vi "Get StartStop Status.vi"(8 "error in":errorcluster, 11 "VISA resource name in":refnum<visa-resource-name>) -> (0 "error out":errorcluster, 1 "Status":bool, 3 "VISA resource name out":refnum<visa-resource-name>)   [LabVIEW 2021, in "JULABO DeviceDriver.lvlib"]
doc: "This VI returns true if the instrument is started or false if it is in Standby-Mode"
uses:
  JULABO DeviceDriver.lvlib
panel:
  out "String (output)":string
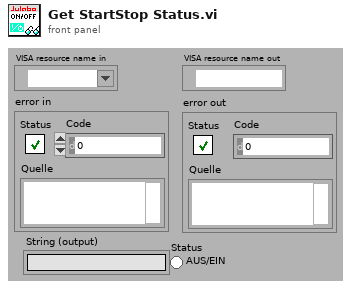
[diagram p1: front panel]
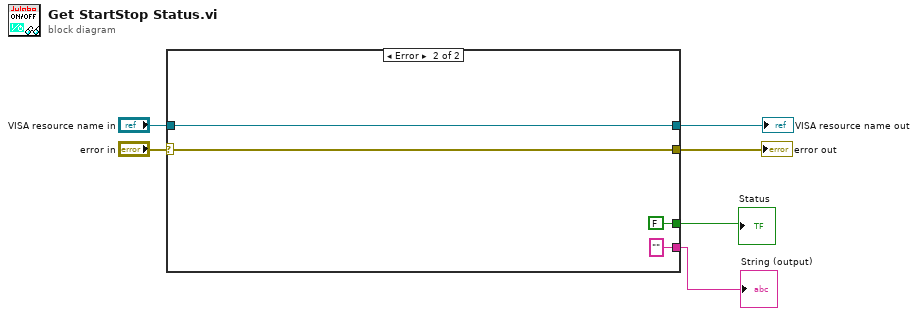
[diagram p0: block diagram]
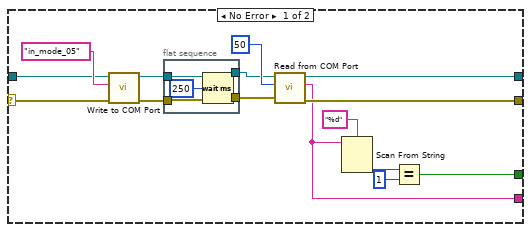
[diagram p2: hidden frame]
diagram:
  n1 = case shown="Error" "error in" {
    selector: "error in" -> [w13 w27]
    tunnel: [w20 w27] -> w6
    tunnel: [w18 w28] -> w5
    tunnel: "VISA resource name in" -> [w16 w28]
    tunnel: [w8 FALSE] -> w2
    tunnel: [w7 "" ("String (output)")] -> w1
    frame No Error {
      n2 = call "Write to COM Port.vi"("error in"=w13, "Command (input)"="in_mode_05", "VISA resource name in"=w16) -> ("error out"=w9:errorcluster, "VISA resource name out"=w11:refnum<visa-resource-name>)  [unwired: 7 in]
      n3 = flat-sequence {
        tunnel: [w23] -> w12
        tunnel: w11 -> [w23]
        tunnel: [w22] -> w10
        tunnel: w9 -> [w22]
        frame #0 {
          n4 = Wait (ms)(milliseconds to wait=u32 250) -> ()  [unwired: 1 out]
        }
      }
      n5 = call "Read from COM Port.vi"("error in"=w10, "Byte to Read (-1:All)"=u32 50 ("Anzahl der Byte"), "VISA resource name in"=w12) -> ("error out"=w20:errorcluster, "String (output)"=w7:string, "VISA resource name out"=w18:refnum<visa-resource-name>)  [unwired: 5 in, 1 out]
      n6 = Scan From String(format string="%d" ("Format-String"), input string=w7) -> (output 1=w15:i32)  [unwired: 3 in, 3 out]
      n7 = Equal?(x=w15, y=1) -> (x = y?=w8:bool)
    }
    frame Error {
    }
  }
  "error out" <- w6
  "VISA resource name out" <- w5
  "Status" <- w2
  "String (output)" <- w1
